vi "FileIOTesting.vi"() -> ()   [LabVIEW 2013]
panel:
  in  "stop":bool
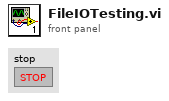
[diagram p1: front panel]
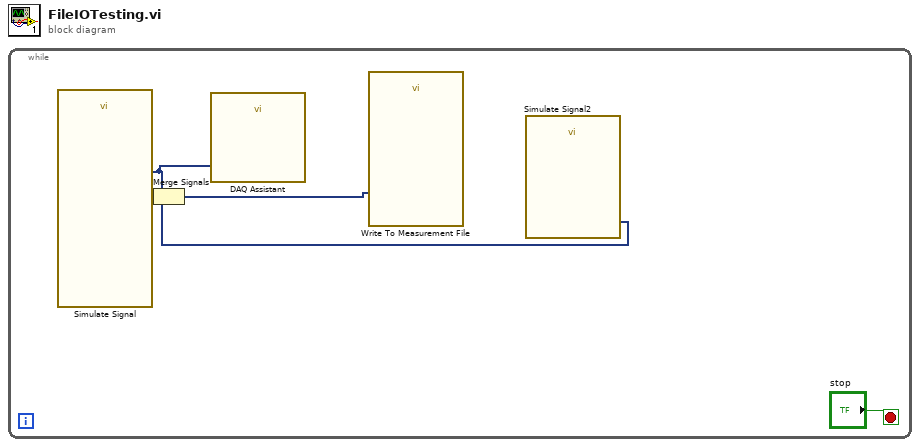
[diagram p0: block diagram]
diagram:
  n1 = while {
    stop <- "stop" stop-if-true
    n2 = call "Simulate Signal"() -> ("Sine"=w3:dynamicdata)  [unwired: 14 in, 1 out]
    n3 = call "DAQ Assistant"("data"=w3) -> ()  [unwired: 17 in, 2 out]
    n4 = call "Simulate Signal2"() -> ("Square"=w1:dynamicdata)  [unwired: 14 in, 1 out]
    n5 = Merge Signals(w3, w1) -> (w2:dynamicdata)
    n6 = call "Write To Measurement File"("Signals"=w2) -> ()  [unwired: 16 in, 3 out]
  }
